vi "Main.vi"   [LabVIEW 2017]
uses:
  Modules/Error/Error.lvlib
  Modules/WebRead/WebRead.lvlib
  Modules/UI/UI.lvlib
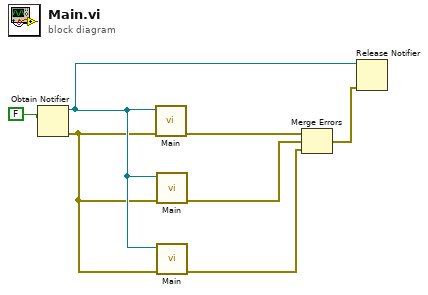
[diagram p0: block diagram]
diagram:
  n1 = Obtain Notifier(notification data type=FALSE) -> (notifier out=w3:refnum<notifier>, error out=w2:errorcluster)  [unwired: 3 in, 1 out]
  n2 = call "Main.vi"("error in (no error)"=w2, "Stop notifier"=w3) -> ("error out"=w6:errorcluster)  [unwired: 9 in]
  n3 = call "Main.vi"("error in (no error)"=w2, "Stop notifier"=w3) -> ("error out"=w5:errorcluster)  [unwired: 9 in]
  n4 = call "Main.vi"("error in (no error)"=w2, "Stop notifier"=w3) -> ("error out"=w1:errorcluster)  [unwired: 9 in]
  n5 = Merge Errors(w6, w5, w1) -> (w4:errorcluster)
  n6 = Release Notifier(notifier=w3, error in (no error)=w4) -> ()  [unwired: 1 in, 3 out]
